vi "Task_code_ASYNCH.vi"(5 "CurrentBufferSize":i32, 6 "SoundWave":waveform(dbl), 7 "CardioSynchExperimentalMatrix":i32[][](array[numeric]), 8 "StimIndice":i16, 9 "Bloc":i8, 10 "TriggerPort":refnum<visa-resource-name>, 11 "AsynchTimeIN":i32) -> (1 "StimIndice_Next":i16, 2 "TriggerPort":refnum<visa-resource-name>, 3 "AsynchTimeOUT":i32)   [LabVIEW 2022 SP3]
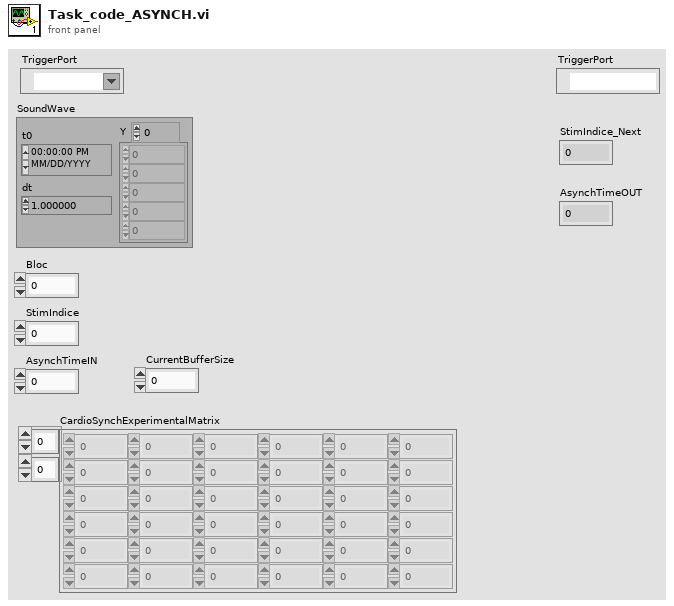
[diagram p1: front panel]
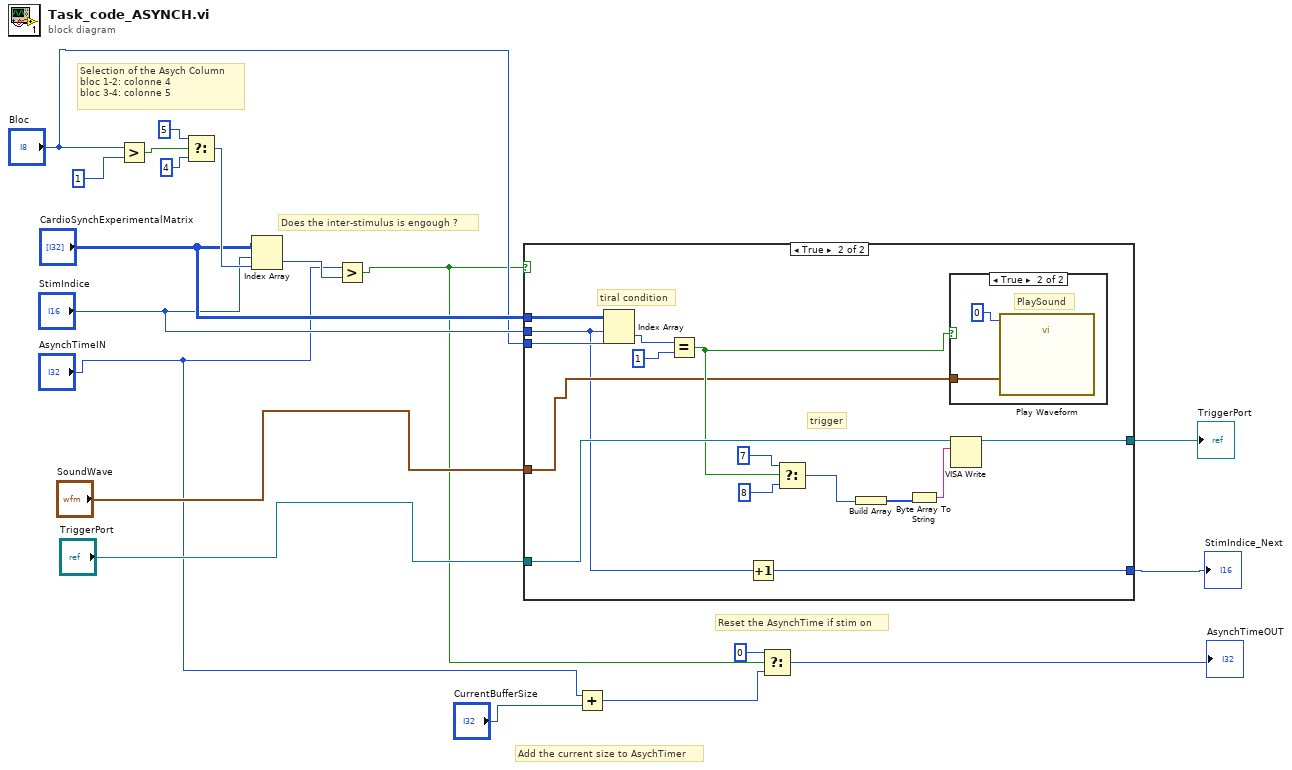
[diagram p0: block diagram]
diagram:
  # "Add the current size to AsychTimer"
  # "Reset the AsynchTime if stim on"
  # "Does the inter-stimulus is engough ?"
  # "Selection of the Asych Column\nbloc 1-2: colonne 4\nbloc 3-4: colonne 5"
  n1 = Greater?(x="Bloc", y=i8 1) -> (0:w14:bool)
  n2 = Select(t=i8 5, s=w14, f=i8 4 ("t")) -> (s? t:f=w11:i8)
  n3 = Index Array(array="CardioSynchExperimentalMatrix", index (row)="StimIndice", index (col)=w11) -> (element=w10:i32)
  n4 = Greater?(x="AsynchTimeIN", y=w10) -> (0:w6:bool)
  n5 = case shown="True" w6 {
    tunnel: "CardioSynchExperimentalMatrix" -> [_ w36]
    tunnel: "StimIndice" -> [w20 w23]
    tunnel: "Bloc" -> [_ w35]
    tunnel: "TriggerPort" -> [w21 w28]
    tunnel: [w21 w27] -> w18
    tunnel: "SoundWave" -> [_ w24]
    tunnel: [w20 w22] -> w16
    frame False {
      # "no R-peak"
    }
    frame True {
      # "trigger"
      # "tiral condition"
      n6 = Index Array(array=w36, index (row)=w23, index (col)=w35) -> (element=w34:i32)
      n7 = Equal?(x=w34, y=1) -> (x = y?=w25:bool)
      n8 = Increment(x=w23) -> (x+1=w22:i16)
      n9 = Select(t=i8 7, s=w25, f=i8 8 ("t")) -> (s? t:f=w26:i8)
      n10 = Build Array(w26) -> (w30:i8[])
      n11 = Byte Array To String(unsigned byte array=w30) -> (string=w29:string)
      n12 = case shown="True" w25 {
        tunnel: w24 -> [_ w37]
        frame False {
        }
        frame True {
          # "PlaySound"
          n13 = call "Play Waveform"("Device"=u32 0, "Data"=w37) -> ()  [unwired: 17 in, 1 out]
        }
      }
      n14 = VISA Write(VISA resource name=w28, write buffer=w29) -> (VISA resource name out=w27:refnum<visa-resource-name>)  [unwired: 1 in, 2 out]
    }
  }
  "TriggerPort" <- w18
  "StimIndice_Next" <- w16
  n15 = Add(x="AsynchTimeIN", y="CurrentBufferSize") -> (x+y=w1:i32)
  n16 = Select(t=0, s=w6, f=w1) -> (s? t:f=→"AsynchTimeOUT":i32)
